vi "configuration_relative.vi"(10 "to_relative":bool, 11 "configuration in":T1) -> (3 "configuration out":T1)   [LabVIEW 2015, in "lv-builder-default.lvlib"]
uses:
  lv-builder-default.lvlib
  public/_controls/configuration.ctl
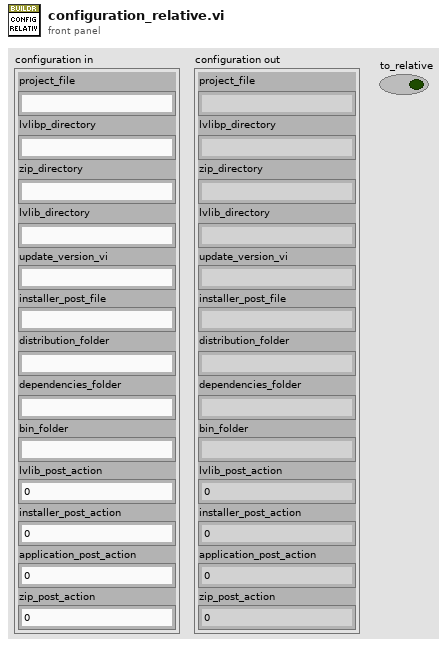
[diagram p1: front panel]
types:
  T1 = typedef "lv-builder-default.lvlib/configuration.ctl" = cluster{"project_file":string, "lvlibp_directory":string, "zip_directory":string, "lvlib_directory":string, "update_version_vi":string, "installer_post_file":string, "distribution_folder":string, "dependencies_folder":string, "bin_folder":string, "lvlib_post_action":u16, "installer_post_action":u16, "application_post_action":u16, "zip_post_action":u16}
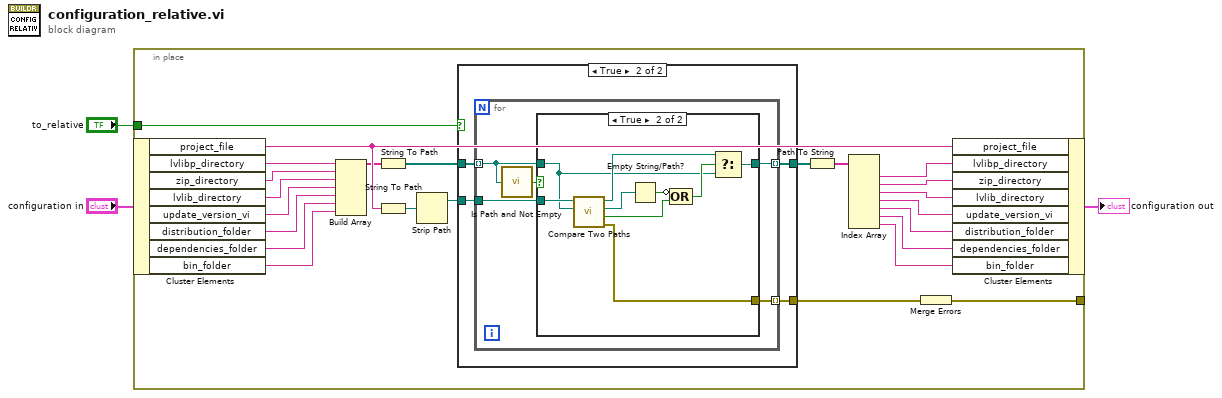
[diagram p0: block diagram]
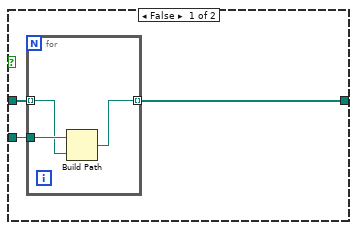
[diagram p2: hidden frame]
diagram:
  n1 = in-place {
    in-place-border: "to_relative" -> [w10]
    in-place-border: [w4] -> _
    n2 = in-place-cluster #1("configuration in") -> ("project_file"=w21:string, "lvlibp_directory"=w27:string, "zip_directory"=w26:string, "lvlib_directory"=w25:string, "update_version_vi"=w24:string, "distribution_folder"=w23:string, "dependencies_folder"=w22:string, "bin_folder"=w7:string)
    n3 = Build Array(w27, w26, w25, w24, w23, w22, w7) -> (w20:string[])
    n4 = String To Path(string=w20) -> (path=w19:path[])
    n5 = String To Path(string=w21) -> (path=w9:path)
    n6 = Strip Path(path=w9) -> (stripped path=w8:path)  [unwired: 1 out]
    n7 = case shown="True" w10 {
      tunnel: w8 -> [w30 w37]
      tunnel: w19 -> [w29 w36]
      tunnel: [w28 w35] -> w18
      tunnel: [_ w34] -> w5
      frame False {
        n8 = for {
          tunnel: w30 -> [w33]
          tunnel: w29 -> [w32] mode=indexing
          tunnel: [w31] -> w28 mode=indexing
          n9 = Build Path(base path=w33, name or relative path=w32) -> (appended path=w31:path)
        }
      }
      frame True {
        n10 = for {
          tunnel: w37 -> [w41]
          tunnel: w36 -> [w40] mode=indexing
          tunnel: [w42] -> w35 mode=indexing
          tunnel: [w38] -> w34 mode=indexing
          n11 = call <vilib>:"Is Path and Not Empty.vi"("path"=w40) -> ("Is Path and Not Empty?"=w39:bool)  [unwired: 4 in]
          n12 = case shown="True" w39 {
            tunnel: [w43 w48] -> w42
            tunnel: [_ w47] -> w38
            tunnel: w41 -> [_ w46]
            tunnel: w40 -> [w43 w44]
            frame False {
            }
            frame True {
              n13 = call <vilib>:"Compare Two Paths.vi"("Path 2"=w44, "Path 1"=w46) -> ("error out"=w47:errorcluster, "Path 2 Relative to Path 1?"=w45:bool, "Common Path"=w52:path, "Relative Path from 1 to 2"=w50:path)  [unwired: 6 in]
              n14 = Empty String/Path?(string/path=w52) -> (empty?=w51:bool)
              n15 = Compound Arithmetic op=OR(invert w51, w45) -> (w49:bool)
              n16 = Select(t=w50, s=w49, f=w44) -> (s? t:f=w48:path)
            }
          }
        }
      }
    }
    n17 = Path To String(path=w18) -> (string=w17:string[])
    n18 = Index Array(array=w17) -> (element #1=w16:string, element #2=w15:string, element #3=w14:string, element #4=w13:string, element #5=w12:string, element #6=w11:string, element #7=w6:string)  [unwired: 7 in]
    n19 = Merge Errors(w5) -> (w4:errorcluster)
    n20 = in-place-cluster #1("project_file"=w21, "lvlibp_directory"=w16, "zip_directory"=w15, "lvlib_directory"=w14, "update_version_vi"=w13, "distribution_folder"=w12, "dependencies_folder"=w11, "bin_folder"=w6) -> (→"configuration out":T1)
  }
